vi "Strategy 3_not the pid.vi"() -> ()   [LabVIEW 2018]
uses:
  <vilib>/DAQmx/write.llb/DAQmx Write (Digital 1D Bool 1Chan 1Samp).vi
  <vilib>/DAQmx/create/channels.llb/DAQmx Create Channel (DO-Digital Output).vi
  <vilib>/DAQmx/miscellaneous.llb/DAQmx Fill In Error Info.vi
  <vilib>/ptbypt/NI_PtbyPt.lvlib
panel:
  in  "Boolean":bool
  in  "sample length":i32=50
  out "Waveform Chart":dbl(graph)
  in  "Set Point":dbl(slide) scale=0.0..40.0
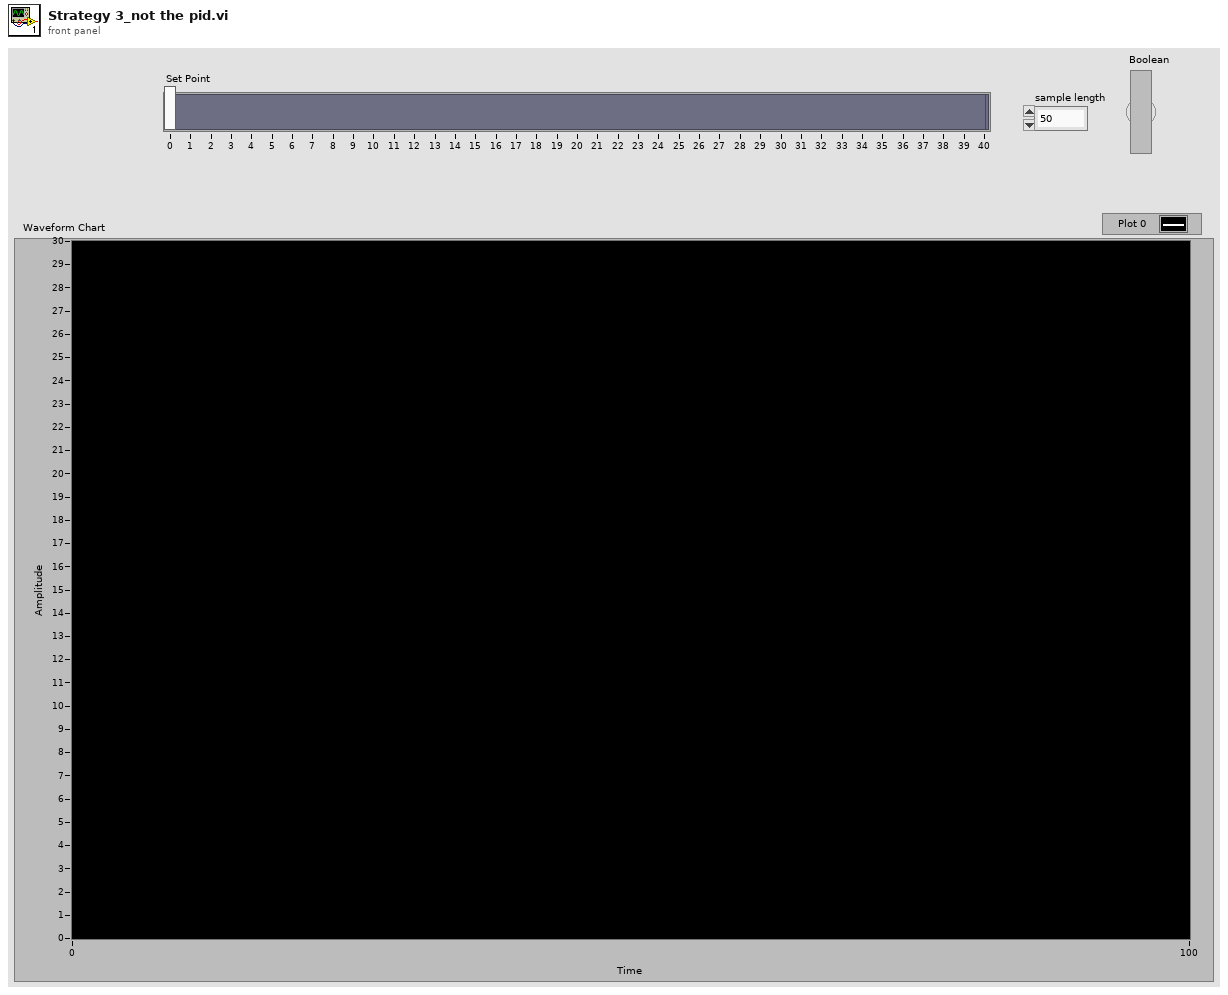
[diagram p1: front panel]
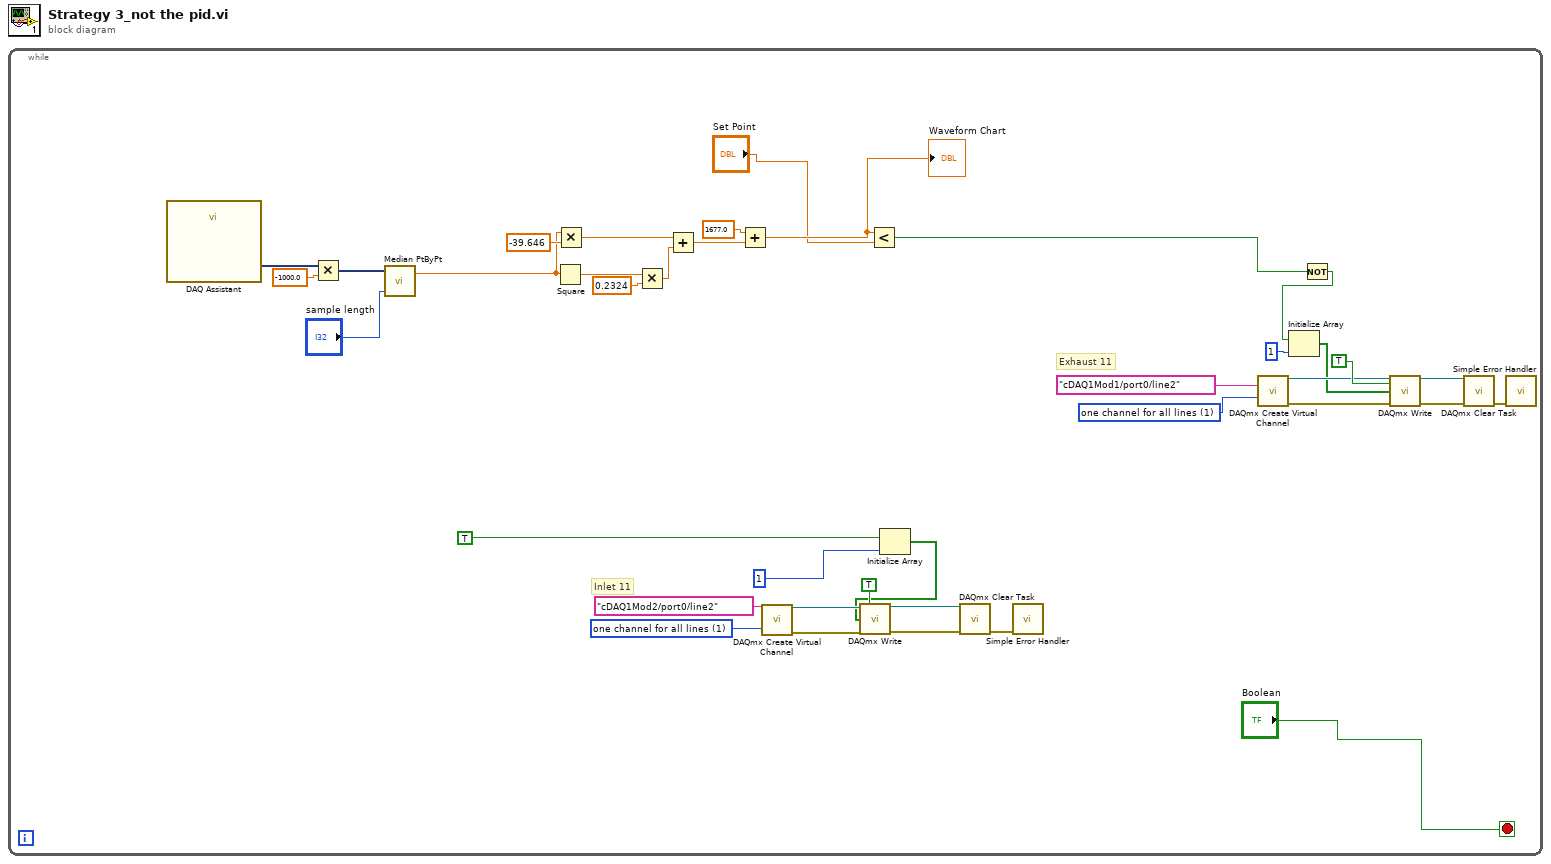
[diagram p0: block diagram]
diagram:
  n1 = while {
    stop <- "Boolean" stop-if-true
    w6 = 1 items=["one channel for each line", "one channel for all lines"] ("line grouping")
    w20 = 1 items=["one channel for each line", "one channel for all lines"] ("line grouping")
    # "Inlet 11"
    # "Exhaust 11"
    n2 = call "DAQ Assistant"() -> ("data"=w38:dynamicdata)  [unwired: 17 in, 2 out]
    n3 = Multiply(x=w38, y=-1000.0) -> (x*y=w29:dynamicdata)
    n4 = call <vilib>:"Median PtByPt.vi"("sample length"="sample length", "x"=w29) -> ("median"=w28:dbl)  [unwired: 2 in, 1 out]
    n5 = Square(x=w28) -> (x^2=w36:dbl)
    n6 = Multiply(x=w28, y=-39.646) -> (x*y=w32:dbl)
    n7 = Multiply(x=w36, y=0.2324) -> (x*y=w33:dbl)
    n8 = Add(x=w32, y=w33) -> (x+y=w31:dbl)
    n9 = Add(x=1677.0, y=w31) -> (x+y=w14:dbl)
    "Waveform Chart" <- w14
    n10 = call-poly <vilib>:"DAQmx Create Virtual Channel.vi"("lines"=tag "cDAQ1Mod2/port0/line2", "line grouping"=w6) -> ("task out"=w8:refnum<k21>, "error out"=w7:errorcluster)  [unwired: 12 in]
    n11 = Less?(x=w14, y="Set Point") -> (x < y?=w16:bool)
    n12 = Initialize Array(TRUE, 1 ("dimension size")) -> (w3:bool[])
    n13 = call-poly <vilib>:"DAQmx Write.vi"("task/channels in"=w8, "auto start"=TRUE, "data"=w3, "error in"=w7) -> ("task out"=w10:refnum<k21>, "error out"=w11:errorcluster)  [unwired: 9 in, 1 out]
    n14 = call <vilib>:"DAQmx Clear Task.vi"("task in"=w10, "error in"=w11) -> ("error out"=w5:errorcluster)  [unwired: 13 in]
    n15 = call <vilib>:"Simple Error Handler.vi"("error in (no error)"=w5) -> ()  [unwired: 4 in, 5 out]
    n16 = call-poly <vilib>:"DAQmx Create Virtual Channel.vi"("lines"=tag "cDAQ1Mod1/port0/line2", "line grouping"=w20) -> ("task out"=w22:refnum<k21>, "error out"=w21:errorcluster)  [unwired: 12 in]
    n17 = Not(x=w16) -> (.not. x?=w15:bool)
    n18 = Initialize Array(w15, 1 ("dimension size")) -> (w17:bool[])
    n19 = call-poly <vilib>:"DAQmx Write.vi"("task/channels in"=w22, "auto start"=TRUE, "data"=w17, "error in"=w21) -> ("task out"=w24:refnum<k21>, "error out"=w25:errorcluster)  [unwired: 9 in, 1 out]
    n20 = call <vilib>:"DAQmx Clear Task.vi"("task in"=w24, "error in"=w25) -> ("error out"=w19:errorcluster)  [unwired: 13 in]
    n21 = call <vilib>:"Simple Error Handler.vi"("error in (no error)"=w19) -> ()  [unwired: 4 in, 5 out]
  }
